vi "Station Overview.vi"() -> ()   [LabVIEW 2015, in "Overview GUI.lvlib"]
uses:
  Overview GUI.lvlib
  Types/Overview.StateVariables.ctl
  <vilib>/NI Veristand/Execution/Workspace/WorkspaceAPI.ctl
  <vilib>/NI Veristand/Execution/Workspace/SystemStateRegEventRef.ctl
  <vilib>/NI Veristand/Execution/Workspace/Target State Info.ctl
  <vilib>/NI Veristand/Execution/Workspace/Target State.ctl
  <vilib>/NI Veristand/Execution/Workspace/SystemStateEventRef.ctl
  <vilib>/NI/AMC/Read Termination Message.vi
  <vilib>/NI/AMC/Update Message Routing Info.vi
  <vilib>/NI/AMC/Create Multiple Messages.vi
  <vilib>/NI/AMC/Create Single Message.vi
  <vilib>/NI/AMC/Globals.vi
  <vilib>/NI/AMC/Send Message.vi
  <vilib>/NI/AMC/AMC.lvlib
  <vilib>/NI Veristand/Execution/Workspace/NI_VS Workspace ExecutionAPI.lvlib
  NationalInstruments.VeriStand.ClientAPI
panel:
  in  "Station.IDs":string[](array[string])=["Station_1"]
  in  "NIVS.Gateway IP Address":string="localhost"
  in  "NIVS.Workspace Event":refnum<event-registration>
  out "Station ID":string
  out "Multicolumn Listbox":i32(listbox)
  in  "Station.ID":string="All"
  in  "exit":bool
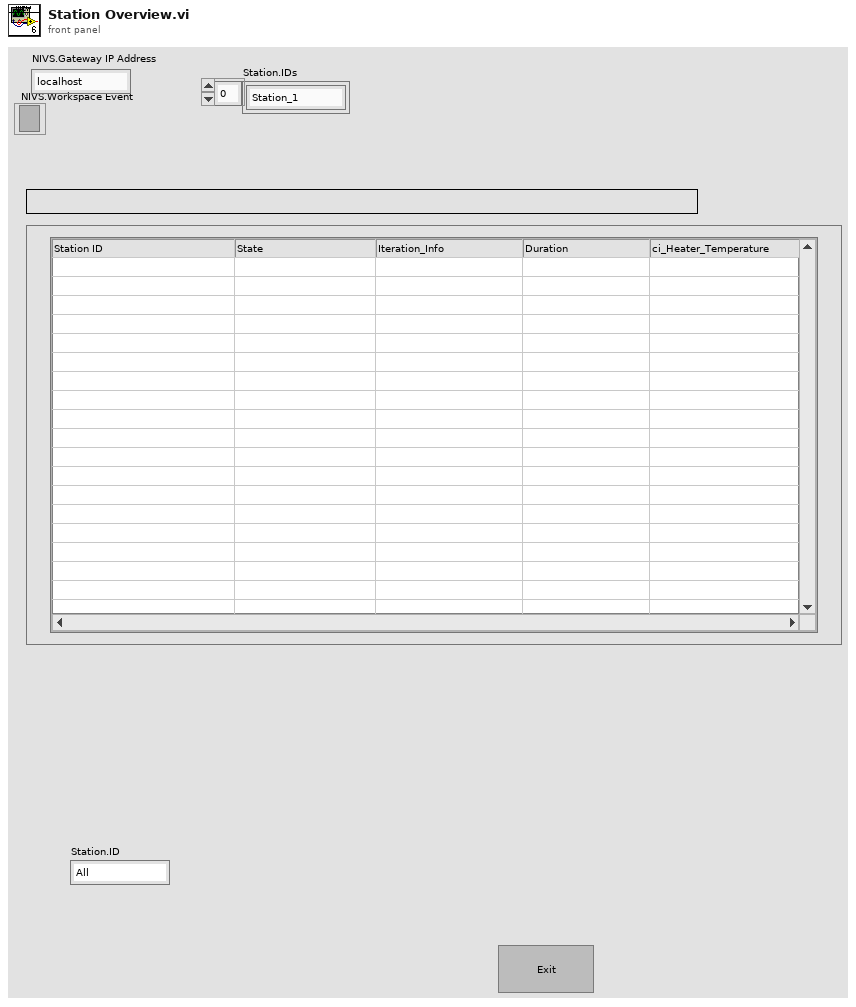
[diagram p1: front panel]
types:
  T1 = typedef "Overview GUI.lvlib/Overview.StateVariables.ctl" = cluster{"UI.Table":refnum<vi>, "NIVS.Gateway IP Address":string, "NIVS.WorkspaceManager":T2, "NIVS.Events":cluster{"SystemChangeEvent":T3, "WorkspaceEvent":refnum<event-registration>}, "NIVS.SystemStateRefs":T4, "NIVS.Deployed":bool, "Channel.List":string[], "Station.IDs":string[], "Counter":u8}
  T2 = typedef "NI_VS Workspace ExecutionAPI.lvlib/WorkspaceAPI.ctl" = refnum<k24>
  T3 = typedef "NI_VS Workspace ExecutionAPI.lvlib/SystemStateRegEventRef.ctl" = refnum<event-registration>
  T4 = typedef "NI_VS Workspace ExecutionAPI.lvlib/SystemStateEventRef.ctl" = cluster{"CustDatRef":refnum<user-event>, "EvtRef":refnum<k27>, "Target State User Event":refnum<user-event>}
  T5 = typedef "AMC.lvlib/Message Queue.ctl" = refnum<queue>
  T6 = cluster{"SystemChangeEvent":T3, "WorkspaceEvent":refnum<event-registration>}
  T7 = typedef "NI_VS Workspace ExecutionAPI.lvlib/SystemState.ctl" = u8
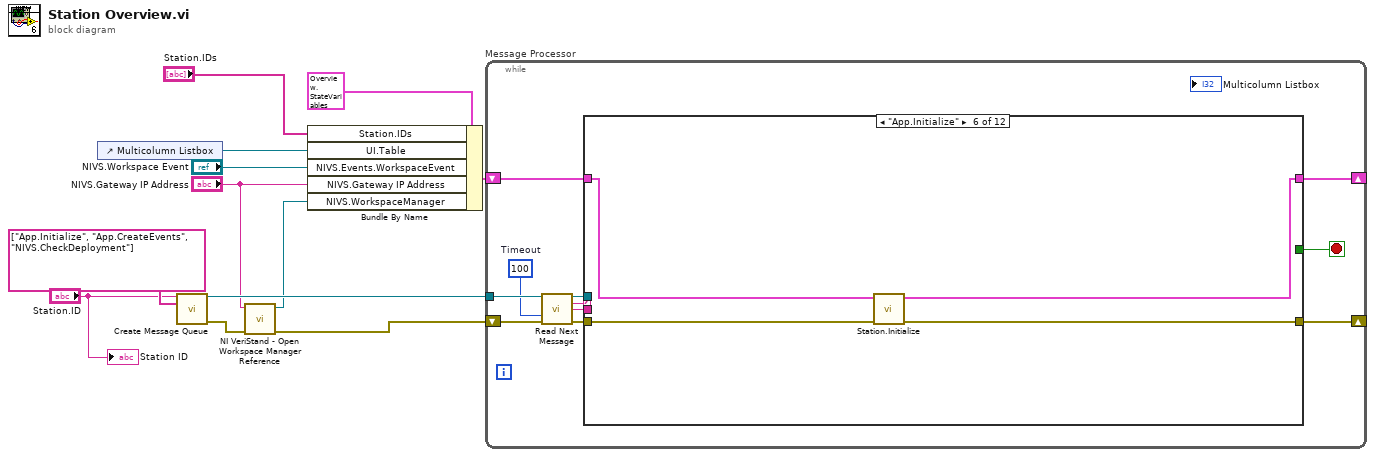
[diagram p0: block diagram]
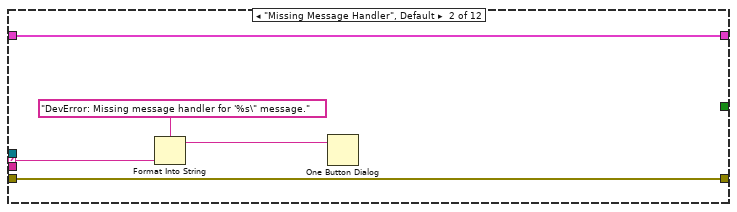
[diagram p3: hidden frame]
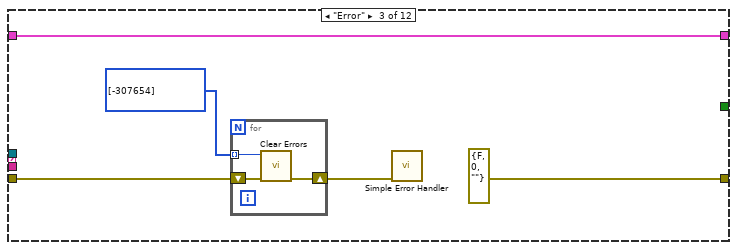
[diagram p4: hidden frame]
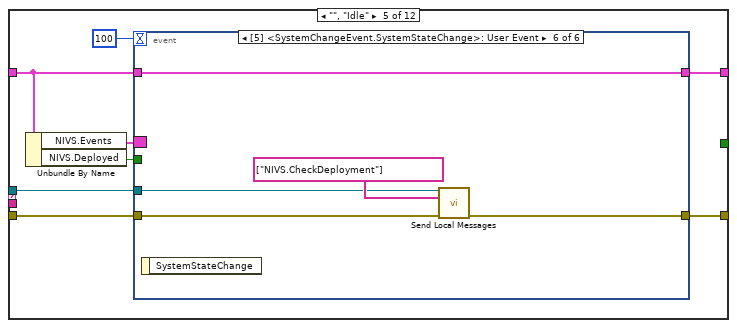
[diagram p6: hidden frame]
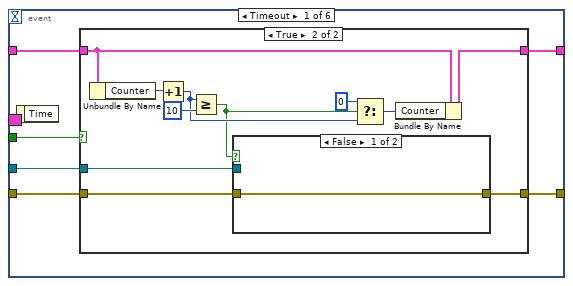
[diagram p7: hidden frame]
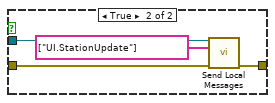
[diagram p9: hidden frame]
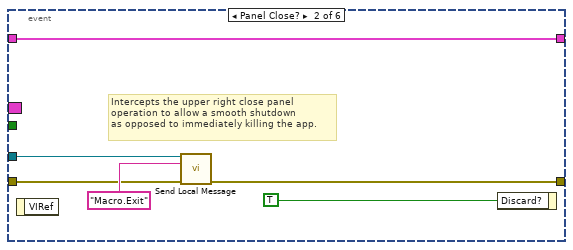
[diagram p10: hidden frame]
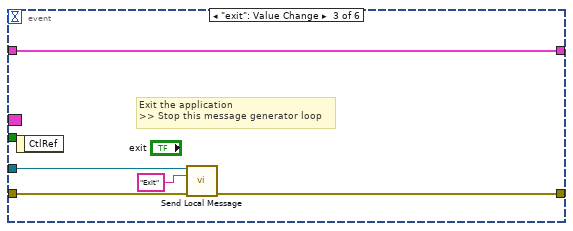
[diagram p11: hidden frame]
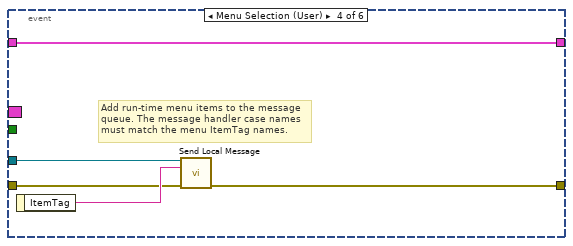
[diagram p12: hidden frame]
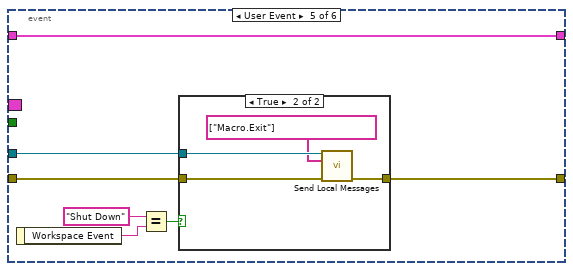
[diagram p13: hidden frame]
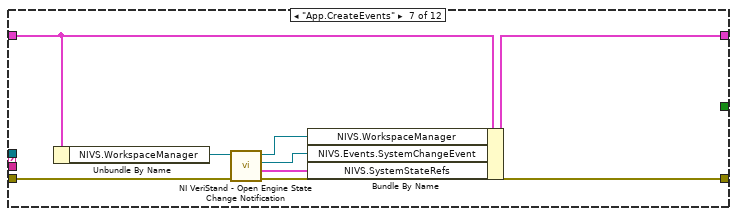
[diagram p15: hidden frame]
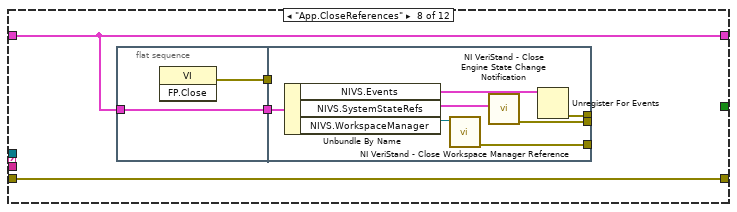
[diagram p16: hidden frame]
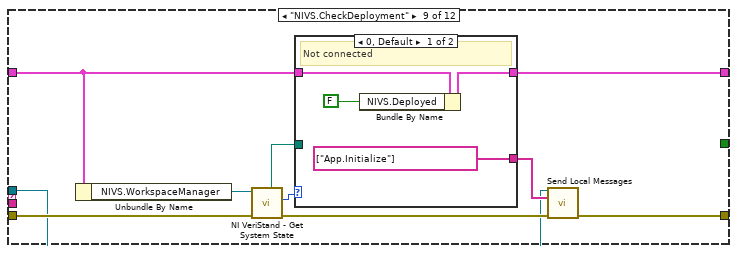
[diagram p17: hidden frame]
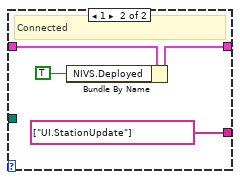
[diagram p18: hidden frame]
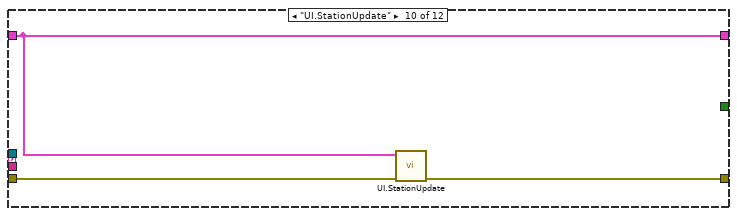
[diagram p19: hidden frame]
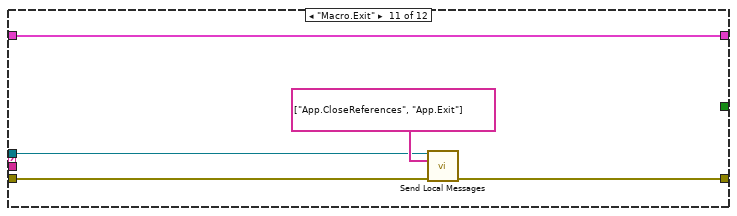
[diagram p20: hidden frame]
diagram:
  n1 = control-ref of="Multicolumn Listbox"() -> (w8:refnum<vi>)
  n2 = call <vilib>:"Create Message Queue.vi"("message queue name"="Station.ID", "initial message names"=string[] ["App.Initialize", "App.CreateEvents", "NIVS.CheckDeployment"]) -> ("message queue out"=w11:T5, "error out"=w7:errorcluster)  [unwired: 12 in]
  n3 = call <vilib>:"NI VeriStand - Open Workspace Manager Reference.vi"("error in (no error)"=w7, "Gateway IP Address (\"\": localhost)"="NIVS.Gateway IP Address") -> ("error out"=w6:errorcluster, "WorkspaceManager"=w3:T2)  [unwired: 8 in]
  n4 = Bundle By Name(cluster=T1 {"UI.Table"=refnum, "NIVS.Gateway IP Address"="", "NIVS.WorkspaceManager"=refnum, "NIVS.Events"={"SystemChangeEvent"=refnum, "WorkspaceEvent"=refnum}, "NIVS.SystemStateRefs"={"CustDatRef"=refnum, "EvtRef"=refnum, "Target State User Event"=refnum}, "NIVS.Deployed"=FALSE, "Channel.List"=[], "Station.IDs"=[], "Counter"=0} ("state variables"), "Station.IDs"="Station.IDs", "UI.Table"=w8, "NIVS.Events.WorkspaceEvent"="NIVS.Workspace Event", "NIVS.Gateway IP Address"="NIVS.Gateway IP Address", "NIVS.WorkspaceManager"=w3) -> (w9:T1)
  n5 = while "Message Processor" {
    shift-left: w6 -> [w18]
    shift-right: [w21] -> _
    tunnel: w11 -> [w19]
    shift-left: w9 -> [w23]
    shift-right: [w22] -> _
    stop <- w13 stop-if-true
    w14 = 100  # Timeout
    n6 = call <vilib>:"Read Next Message.vi"("message queue in"=w19, "timeout (1 ms)"=w14, "error in"=w18) -> ("message queue out"=w20:T5, "message name"=w16:string, "message value"=w15:string, "error out"=w17:errorcluster)  [unwired: 5 in, 4 out]
    n7 = case shown="\"App.Initialize\"" w16 {
      selector: w16 -> [_ w28 _ _ _ _ _ _ _ _ _ _]
      tunnel: [w25 w30 w35 w40 w41 w108 w113 w120 w132 w149 w156 w161] -> w22
      tunnel: w23 -> [w25 w30 w35 w40 w42 w109 w112 w120 w133 w149 w156 w161]
      tunnel: w20 -> [_ _ _ _ w48 _ _ _ w134 _ w152 w159]
      tunnel: w17 -> [w24 w29 w31 w39 w47 w107 w117 w121 w135 w151 w154 w160]
      tunnel: [w24 w29 errorcluster {"status"=FALSE, "code"=0, "source"=""} ("error out") w39 w46 w106 w116 w121 w131 w150 w153 w158] -> w21
      tunnel: w15 -> [_ _ _ _ _ _ _ _ _ _ _ _]
      tunnel: [_ _ _ _ _ _ _ _ _ _ _ TRUE] -> w13
      frame "---------- Framework Operations ----------" {
      }
      frame "Missing Message Handler", Default {
        n8 = Format Into String(format string="DevError: Missing message handler for '%s\" message." ("message"), w28) -> (resulting string=w26:string)  [unwired: 2 in, 1 out]
        n9 = One Button Dialog(message=w26) -> ()  [unwired: 2 out]
      }
      frame "Error" {
        n10 = for {
          shift-right: [w37] -> w32
          shift-left: w31 -> [w38]
          tunnel: i32[] [-307654] -> [w36] mode=indexing
          n11 = call <vilib>:"Clear Errors.vi"("error in (no error)"=w38, "specific error code to clear (0: all)"=w36) -> ("error out"=w37:errorcluster)  [unwired: 4 in, 1 out]
        }
        n12 = call <vilib>:"Simple Error Handler.vi"("error in (no error)"=w32) -> ()  [unwired: 1 in, 8 out]
      }
      frame "---------- Application Operations ----------" {
      }
      frame "", "Idle" {
        n13 = Unbundle By Name(w42) -> ("NIVS.Events"=w45:T6, "NIVS.Deployed"=w43:bool)
        n14 = event shown="[5] <SystemChangeEvent.SystemStateChange>: User Event" {
          selector: w45 -> [_ _ _ _ _ _]
          dyn-events: _ -> [_ _ _ _ _ _]
          timeout: 100 -> [_ _ _ _ _ _]
          tunnel: w48 -> [w54 w76 w82 w87 w92 w103]
          tunnel: w47 -> [w53 w75 w81 w86 w93 w104]
          tunnel: [w52 w74 w80 w85 w91 w102] -> w46
          tunnel: w43 -> [w51 _ _ _ _ _]
          tunnel: w42 -> [w50 w73 w79 w84 w90 w101]
          tunnel: [w49 w73 w79 w84 w90 w101] -> w41
          event Timeout {
            n15 = event-data() -> ()  [unwired: 2 out]
            n16 = case shown="True" w51 {
              tunnel: w54 -> [_ w67]
              tunnel: w53 -> [w56 w66]
              tunnel: [w56 w65] -> w52
              tunnel: w50 -> [w55 w64]
              tunnel: [w55 w58] -> w49
              frame False {
              }
              frame True {
                n17 = Unbundle By Name(w64) -> ("Counter"=w63:u8)
                n18 = Increment(x=w63) -> (x+1=w61:u8)
                n19 = Greater Or Equal?(x=w61, y=u8 10) -> (x >= y?=w57:bool)
                n20 = case shown="False" w57 {
                  tunnel: w67 -> [_ w72]
                  tunnel: w66 -> [w68 w71]
                  tunnel: [w68 w70] -> w65
                  frame False {
                  }
                  frame True {
                    n21 = call <vilib>:"Send Local Messages.vi"("message queue in"=w72, "message names"=string[] ["UI.StationUpdate"], "error in"=w71) -> ("error out"=w70:errorcluster)  [unwired: 10 in, 2 out]
                  }
                }
                n22 = Select(t=u8 0, s=w57, f=w61) -> (s? t:f=w59:u8)
                n23 = Bundle By Name(cluster=w64, "Counter"=w59) -> (w58:T1)
              }
            }
          }
          event Panel Close? {
            # "Intercepts the upper right close panel\noperation to allow a smooth shutdown\nas opposed to immediately killing the app."
            n24 = event-data() -> ()  [unwired: 2 out]
            n25 = call <vilib>:"Send Local Message.vi"("message queue in"=w76, "message name"="Macro.Exit", "error in"=w75) -> ("error out"=w74:errorcluster)  [unwired: 10 in, 2 out]
            n26 = event-data("Discard?"=TRUE) -> ()  [unwired: 1 in, 1 out]
          }
          event "exit": Value Change {
            # "Exit the application\n>> Stop this message generator loop"
            n27 = event-data() -> ()  [unwired: 2 out]
            n28 = call <vilib>:"Send Local Message.vi"("message queue in"=w82, "message name"="Exit", "error in"=w81) -> ("error out"=w80:errorcluster)  [unwired: 10 in, 2 out]
          }
          event Menu Selection (User) {
            # "Add run-time menu items to the message\nqueue. The message handler case names must match the menu ItemTag names."
            n29 = event-data() -> ("ItemTag"=w88:string)  [unwired: 1 out]
            n30 = call <vilib>:"Send Local Message.vi"("message queue in"=w87, "message name"=w88, "error in"=w86) -> ("error out"=w85:errorcluster)  [unwired: 10 in, 2 out]
          }
          event User Event {
            n31 = event-data() -> ("Workspace Event"=w89:string)  [unwired: 1 out]
            n32 = Equal?(x="Shut Down" ("y"), y=w89) -> (x = y?=w94:bool)
            n33 = case shown="True" w94 {
              tunnel: w93 -> [w96 w100]
              tunnel: [w96 w99] -> w91
              tunnel: w92 -> [_ w98]
              frame False {
              }
              frame True {
                n34 = call <vilib>:"Send Local Messages.vi"("message queue in"=w98, "message names"=string[] ["Macro.Exit"], "error in"=w100) -> ("error out"=w99:errorcluster)  [unwired: 10 in, 2 out]
              }
            }
          }
          event User Event {
            n35 = event-data() -> ()  [unwired: 2 out]
            n36 = call <vilib>:"Send Local Messages.vi"("message queue in"=w103, "message names"=string[] ["NIVS.CheckDeployment"], "error in"=w104) -> ("error out"=w102:errorcluster)  [unwired: 10 in, 2 out]
          }
        }
      }
      frame "App.Initialize" {
        n37 = call "Station.Initialize.vi"("error in (no error)"=w107, "state variables in"=w109) -> ("error out"=w106:errorcluster, "state variables out"=w108:T1)  [unwired: 8 in]
      }
      frame "App.CreateEvents" {
        n38 = Unbundle By Name(w112) -> ("NIVS.WorkspaceManager"=w111:T2)
        n39 = call <vilib>:"NI VeriStand - Open Engine State Change Notification.vi"("error in (no error)"=w117, "WorkspaceManager in"=w111) -> ("error out"=w116:errorcluster, "SystemStateRefs"=w115:T4, "SystemChangeEventRef"=w114:T3, "WorkspaceManager out"=w110:T2)  [unwired: 6 in]
        n40 = Bundle By Name(cluster=w112, "NIVS.WorkspaceManager"=w110, "NIVS.Events.SystemChangeEvent"=w114, "NIVS.SystemStateRefs"=w115) -> (w113:T1)
      }
      frame "App.CloseReferences" {
        n41 = flat-sequence {
          tunnel: w120 -> [w123]
          tunnel: [w123] -> w119
          tunnel: [w122] -> w118
          tunnel: [w127] -> _
          tunnel: [w126] -> _
          tunnel: [w125] -> _
          tunnel: w119 -> [w124]
          tunnel: w118 -> [_]
          frame #0 {
            n42 = invoke class="VI" method="FP.Close"() -> (error out=w122:errorcluster)  [unwired: 3 in, 2 out]
          }
          frame #1 {
            n43 = Unbundle By Name(w124) -> ("NIVS.Events"=w130:T6, "NIVS.SystemStateRefs"=w129:T4, "NIVS.WorkspaceManager"=w128:T2)
            n44 = call <vilib>:"NI VeriStand - Close Workspace Manager Reference.vi"("WorkspaceManager"=w128) -> ("error out"=w125:errorcluster)  [unwired: 10 in]
            n45 = call <vilib>:"NI VeriStand - Close Engine State Change Notification.vi"("SystemStateRefs"=w129) -> ("error out"=w126:errorcluster)  [unwired: 10 in]
            n46 = Unregister For Events(event registration refnum=w130) -> (error out=w127:errorcluster)  [unwired: 1 in]
          }
        }
      }
      frame "NIVS.CheckDeployment" {
        n47 = Unbundle By Name(w133) -> ("NIVS.WorkspaceManager"=w137:T2)
        n48 = call <vilib>:"NI VeriStand - Get System State.vi"("error in (no error)"=w135, "WorkspaceManager in"=w137) -> ("error out"=w139:errorcluster, "System State"=w136:T7, "System Definition File"=w138:path)  [unwired: 5 in, 2 out]
        n49 = case shown="0, Default" w136 {
          tunnel: w133 -> [w144 w148]
          tunnel: [w143 w146] -> w132
          tunnel: w138 -> [_ _]
          tunnel: [string[] ["App.Initialize"] string[] ["UI.StationUpdate"]] -> w140
          frame 0, Default {
            # "Not connected"
            n50 = Bundle By Name(cluster=w144, "NIVS.Deployed"=FALSE ("Connected")) -> (w143:T1)
          }
          frame 1 {
            # "Connected"
            n51 = Bundle By Name(cluster=w148, "NIVS.Deployed"=TRUE ("Connected")) -> (w146:T1)
          }
        }
        n52 = call <vilib>:"Send Local Messages.vi"("message queue in"=w134, "message names"=w140, "error in"=w139) -> ("error out"=w131:errorcluster)  [unwired: 10 in, 2 out]
      }
      frame "UI.StationUpdate" {
        n53 = call "UI.StationUpdate.vi"("error in (no error)"=w151, "state variables"=w149) -> ("error out"=w150:errorcluster)  [unwired: 9 in]
      }
      frame "Macro.Exit" {
        n54 = call <vilib>:"Send Local Messages.vi"("message queue in"=w152, "message names"=string[] ["App.CloseReferences", "App.Exit"], "error in"=w154) -> ("error out"=w153:errorcluster)  [unwired: 10 in, 2 out]
      }
      frame "App.Exit" {
        n55 = call <vilib>:"Destroy Message Queue.vi"("message queue in"=w159, "error in"=w160) -> ("error out"=w158:errorcluster)  [unwired: 11 in, 2 out]
      }
    }
  }
  "Station ID" <- "Station.ID"
